vi "MEScope_ZeroCalOhms.vi"(8 "error in":errorcluster) -> (0 "error out":errorcluster, 3 "Return Code":i32)   [LabVIEW 2015]
doc: "MEScope_ZeroCalOhms\n\nDescription:\nThis function will cycle through the resistance scales for Ohms, and read the G16 ADC offsets. The values are stored in the Local EEPROM structure.\nDetail:\nint MEScope_ZeroCalOhms (\nvoid\n);\n\nParameters:\nNone\n\nReturn Values:\nThis function returns a 0 if the function completed successfully. A non-zero return code will indicate error. \nRemarks:\naMEScope_ZeroCalOhms\n\nDescription:\nThis function will cycle through the resistance scales for Ohms, and read the G16 ADC offsets. The values are stored in the Local EEPROM structure.\nDetail:\nint MEScope_ZeroCalOhms (\nvoid\n);\n\nParameters:\nNone\n\nReturn Values:\nThis function returns a 0 if the function completed successfully. A non-zero return code will indicate error. \nRemarks:\n\nSerial Command packet: \nn/a"
uses:
  ScannerDiagDLL.dll
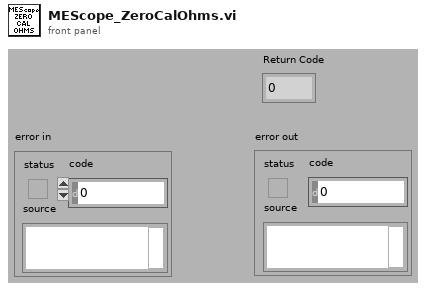
[diagram p1: front panel]
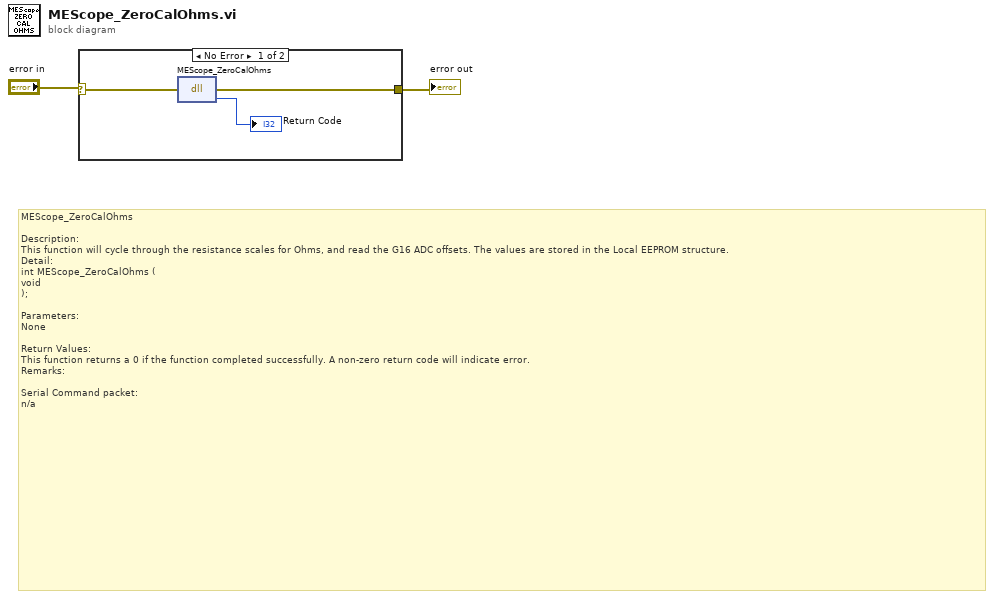
[diagram p0: block diagram]
diagram:
  # "MEScope_ZeroCalOhms\n\nDescription:\nThis function will cycle through the resistance scales for Ohms, and read the G16 ADC offsets. The values are stored in the Local EEPROM structure.\nDetail:\nint MEScope_ZeroCalOhms (\nvoid\n);\n\nParameters:\nNone\n\nReturn Values:\nThis function returns a 0 if the function completed successfully. A non-zero return code will indicate error. \nRemarks:\n\nSerial Command packet: \nn/a"
  n1 = case shown="No Error" "error in" {
    selector: "error in" -> [w4 w6]
    tunnel: [w3 w6] -> w1
    frame No Error {
      n2 = dll-call lib="C:/ModisEdge/TabletScope/Test Sequence/Code Modules/DLL/ScannerDiagDLL.dll" fn="MEScope_ZeroCalOhms"(error in=w4) -> (error out=w3:errorcluster, "return type"=→"Return Code":i32)  [unwired: 2 in, 1 out]
    }
    frame Error {
    }
  }
  "error out" <- w1
